vi "Change Engine Library Placeholders in project.vi"(8 "error in (no error)":errorcluster, 10 "Project Name":string, 11 "Project file content in":string[](array[string])) -> (0 "error out":errorcluster, 3 "Project file content out":string[](array[string]))   [LabVIEW 2019, in "NIVS_Consolidated_CDW_MetaDataObj.lvclass"]
uses:
  NIVS_Consolidated_CDW_MetaDataObj.lvclass
  CD Engine lvlib.ctl
  CD Engine lvlib.vi
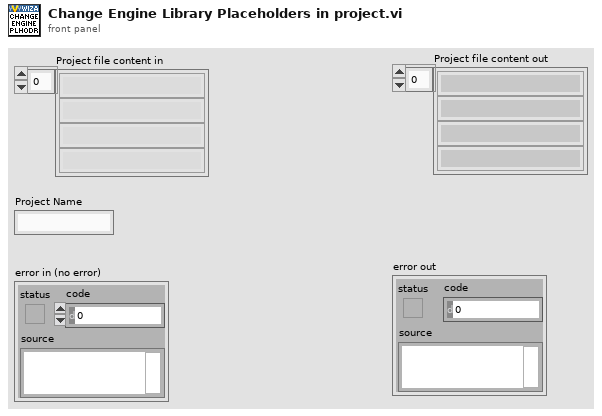
[diagram p1: front panel]
types:
  T1 = typedef "NIVS_Consolidated_CDW_MetaDataObj.lvclass/CD Engine lvlib.ctl" = enum16{"LibraryFileName", "LibraryFolderName", "Engine.FolderName", "Engine.Init.FolderName", "Engine.Run.FolderName", "Engine.Shutdown.FolderName", "Types.FolderName", "Engine.RT Driver VI.TemplatePath", "Engine.RT Driver VI.FileName", "Engine.RTStateVariables.Name", "Engine.RTStateVariables.Name.NoExtension", "Engine.Async.NameExtension", "Engine.Async.TemplateName"}
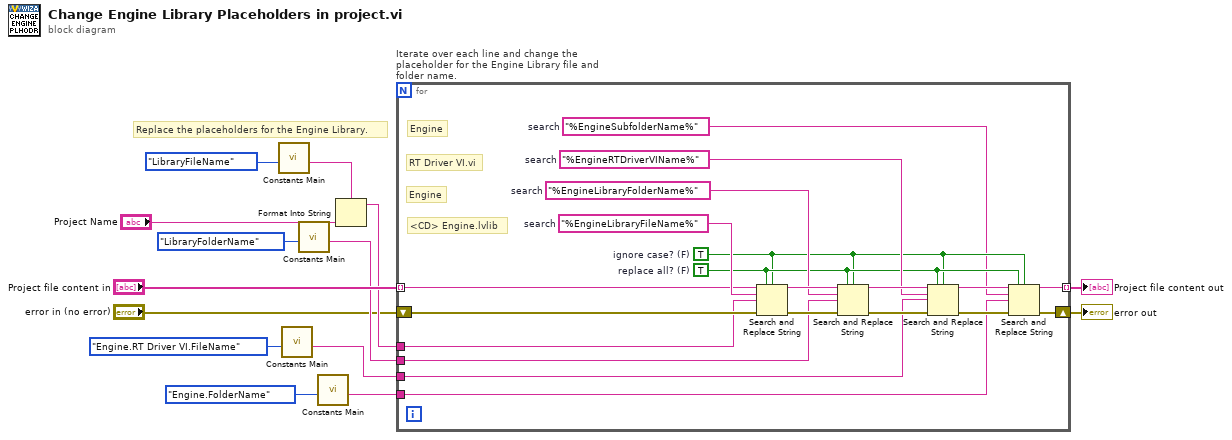
[diagram p0: block diagram]
diagram:
  # "Replace the placeholders for the Engine Library."
  n1 = call-poly "Constants Main.vi"("Action"=CD_Engine_lvlib."LibraryFileName") -> ("Output"=w11:string)  [unwired: 10 in]
  n2 = call-poly "Constants Main.vi"("Action"=CD_Engine_lvlib."Engine.RT Driver VI.FileName") -> ("Output"=w4:string)  [unwired: 10 in]
  n3 = call-poly "Constants Main.vi"("Action"=CD_Engine_lvlib."LibraryFolderName") -> ("Output"=w5:string)  [unwired: 10 in]
  n4 = call-poly "Constants Main.vi"("Action"=CD_Engine_lvlib."Engine.FolderName") -> ("Output"=w3:string)  [unwired: 10 in]
  n5 = Format Into String(format string=w11, "Project Name") -> (resulting string=w6:string)  [unwired: 2 in, 1 out]
  n6 = for "Iterate over each line and change the placeholder for the Engine Library file and folder name." {
    tunnel: "Project file content in" -> [w33] mode=indexing
    shift-right: [w24] -> w14
    shift-left: "error in (no error)" -> [w19]
    tunnel: [w25] -> w13 mode=indexing
    tunnel: w6 -> [w18]
    tunnel: w5 -> [w17]
    tunnel: w4 -> [w16]
    tunnel: w3 -> [w15]
    w23 = "%EngineSubfolderName%"  # search
    w29 = "%EngineRTDriverVIName%"  # search
    w31 = "%EngineLibraryFolderName%"  # search
    w26 = TRUE  # ignore case? (F)
    w27 = TRUE  # replace all? (F)
    w34 = "%EngineLibraryFileName%"  # search
    # "Engine"
    # "RT Driver VI.vi"
    # "Engine"
    # "<CD> Engine.lvlib"
    n7 = Search and Replace String(replace all?=w27, case sensitive?=w26, input string=w33, search string=w34, replace string=w18, error in=w19) -> (result string=w32:string, error out=w21:errorcluster)  [unwired: 2 in, 2 out]
    n8 = Search and Replace String(replace all?=w27, case sensitive?=w26, input string=w32, search string=w31, replace string=w17, error in=w21) -> (result string=w30:string, error out=w20:errorcluster)  [unwired: 2 in, 2 out]
    n9 = Search and Replace String(replace all?=w27, case sensitive?=w26, input string=w30, search string=w29, replace string=w16, error in=w20) -> (result string=w28:string, error out=w22:errorcluster)  [unwired: 2 in, 2 out]
    n10 = Search and Replace String(replace all?=w27, case sensitive?=w26, input string=w28, search string=w23, replace string=w15, error in=w22) -> (result string=w25:string, error out=w24:errorcluster)  [unwired: 2 in, 2 out]
  }
  "error out" <- w14
  "Project file content out" <- w13
